vi "Status Log and Error Handling.vi"(7 "Status Log":refnum<file>, 8 "error in":errorcluster, 10 "Current Bus Number":i32, 11 "Queue in":refnum<queue>) -> (0 "error out":errorcluster, 1 "Current Status":string, 2 "Next State":T1, 3 "Queue out":refnum<queue>, 4 "Status Log":refnum<file>)   [LabVIEW 2014, in "Initialization and IO Node Scripting.lvlib"]
uses:
  Initialization and IO Node Scripting.lvlib
  Scripting States.ctl
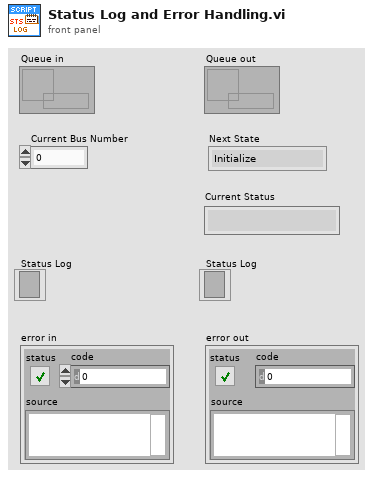
[diagram p1: front panel]
types:
  T1 = typedef "Scripting States.ctl" = enum16{"Initialize", "Copy Template Bus Directory", "Modify Dequeue Commands", "Modify Enqueue Data", "Create FPGA VI", "Create Project FIFOs", "Create FPGA Data Nodes", "Place FPGA Data Nodes", "Update Node Count in Engine", "Expand FIFO Type Def", "Populate FIFO Names in Engine", "Modify I/O Pin Names", "Modify I/O Pin Enable", "Replace DLU", "Add Engine to Project", "Place SPI Engine", "Scripting Complete Check", "End"}
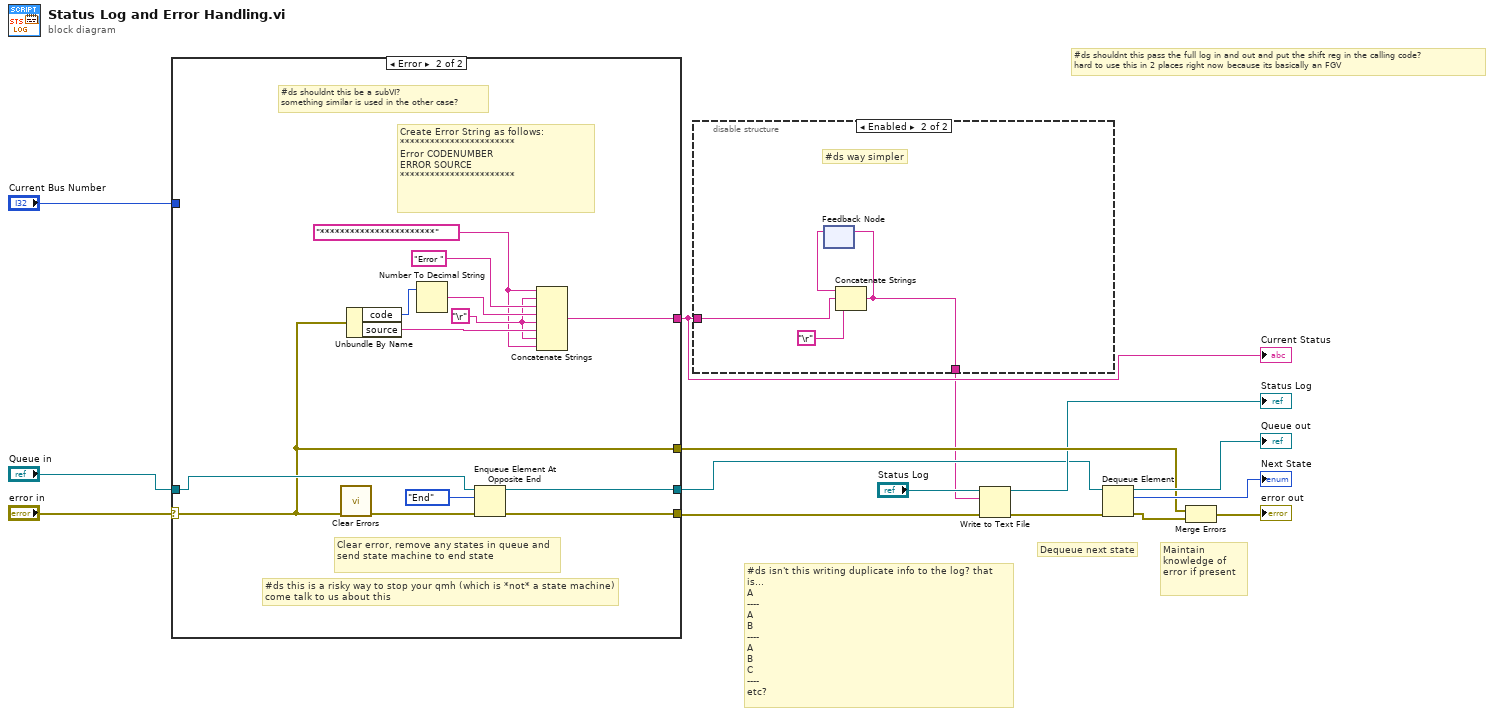
[diagram p0: block diagram]
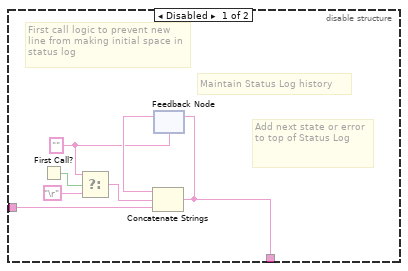
[diagram p2: hidden frame]
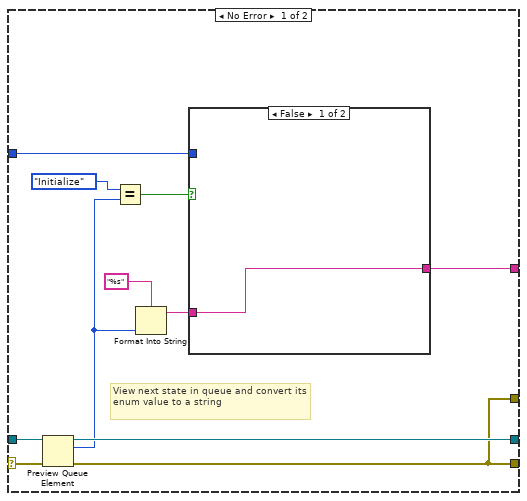
[diagram p3: hidden frame]
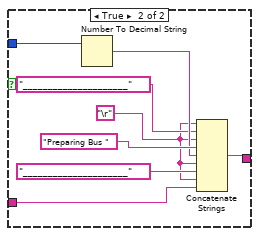
[diagram p4: hidden frame]
diagram:
  # "#ds isn't this writing duplicate info to the log? that is...\nA\n----\nA\nB\n----\nA\nB\nC\n----\netc?"
  # "#ds shouldnt this pass the full log in and out and put the shift reg in the calling code?\nhard to use this in 2 places right now because its basically an FGV"
  # "Maintain knowledge of error if present"
  # "Dequeue next state"
  n1 = case shown="Error" "error in" {
    selector: "error in" -> [w26 w36]
    tunnel: [w18 w45] -> w7
    tunnel: "Queue in" -> [w25 w41]
    tunnel: [w16 w37] -> w6
    tunnel: [w24 w43] -> w2
    tunnel: "Current Bus Number" -> [w20 _]
    tunnel: [w16 w36] -> w8
    frame No Error {
      # "View next state in queue and convert its enum value to a string"
      n2 = Preview Queue Element(queue=w25, error in (no error)=w26) -> (queue out=w24:refnum<queue>, element=w22:T1, error out=w16:errorcluster)  [unwired: 1 in, 1 out]
      n3 = Equal?(x=Scripting_States."Initialize" ("element"), y=w22) -> (x = y?=w19:bool)
      n4 = Format Into String "Format Into String"(format string="%s", w22) -> (resulting string=w17:string)  [unwired: 2 in, 1 out]
      n5 = case shown="False" w19 {
        tunnel: w20 -> [_ w35]
        tunnel: [w27 w34] -> w18
        tunnel: w17 -> [w27 w29]
        frame False {
        }
        frame True {
          w28 = "\r"
          n6 = Number To Decimal String(number=w35) -> (decimal integer string=w32:string)  [unwired: 1 in]
          n7 = Concatenate Strings(w28, "_____________________" ("string"), w28, "Preparing Bus " ("string"), w32, w28, "_____________________" ("string"), w28, w29) -> (w34:string)
        }
      }
    }
    frame Error {
      w38 = "***********************" ("string")
      w39 = "\r"
      # "#ds this is a risky way to stop your qmh (which is *not* a state machine)\ncome talk to us about this"
      # "#ds shouldnt this be a subVI?\nsomething similar is used in the other case?"
      # "Create Error String as follows:\n***********************\nError CODENUMBER\nERROR SOURCE\n***********************"
      # "Clear error, remove any states in queue and send state machine to end state"
      n8 = call <vilib>:"Clear Errors.vi"("error in (no error)"=w36) -> ("error out"=w42:errorcluster)  [unwired: 5 in, 1 out]
      n9 = Unbundle By Name(w36) -> ("code"=w46:i32, "source"=w48:string)
      n10 = Number To Decimal String(number=w46) -> (decimal integer string=w47:string)  [unwired: 1 in]
      n11 = Enqueue Element At Opposite End(queue=w41, element=Scripting_States."End", error in (no error)=w42) -> (queue out=w43:refnum<queue>, error out=w37:errorcluster)  [unwired: 1 in, 1 out]
      n12 = Concatenate Strings(w38, w39, "Error " ("string"), w47, w39, w48, w39, w38) -> (w45:string)
    }
  }
  "Current Status" <- w7
  n13 = disable-structure shown="Enabled" {
    disable-tunnel: w7 -> [w50 w59]
    disable-tunnel: [w49 w56] -> w1
    frame Disabled {
      w51 = ""
      # "Add next state or error to top of Status Log"
      # "Maintain Status Log history"
      # "First call logic to prevent new line from making initial space in status log"
      n14 = First Call?() -> (First Call?: T/F=w52:bool)
      n15 = Select(t=w51, s=w52, f="\r") -> (s? t:f=w53:string)
      n16 = feedback #1(w51) -> (w55:string)
      n17 = Concatenate Strings(w55, w53, w50) -> (w49:string)
      n18 = feedback-in #1(w49) -> ()
    }
    frame Enabled {
      # "#ds way simpler"
      n19 = feedback #2() -> (w58:string)  [unwired: 1 in]
      n20 = Concatenate Strings(w58, w59, "\r") -> (w56:string)
      n21 = feedback-in #2(w56) -> ()
    }
  }
  n22 = Write to Text File(file (use dialog)="Status Log", text=w1, error in=w6) -> (refnum out=→"Status Log":refnum<file>, error out=w3:errorcluster)  [unwired: 1 in, 1 out]
  n23 = Dequeue Element(queue=w2, error in (no error)=w3) -> (queue out=→"Queue out":refnum<queue>, element=→"Next State":T1, error out=w10:errorcluster)  [unwired: 1 in, 1 out]
  n24 = Merge Errors(w8, w10) -> (→"error out":errorcluster)
